vi "SubVI.vi"(5 "Durchläufegesamt":i32, 6 "Array 2":string[](array[string])=array[20229 elements], 10 "search String":string=".vi") -> (0 "Numerisches Element":i32, 2 "#found":i32, 3 "Array":string[](array[string]), 4 "work done analyse":dbl(slide) scale=0.0..100.0)   [LabVIEW 2009]
panel:
  out "search":string[](array[string])
  out "found":string[](array[string])
  out "Array 7":i32[](array[numeric])
  out "Array 6":string[](array[string])
  out "Array 5":bool[](array[boolean])
  out "zwischenerg":string[](array[string])
  out "Array 3":bool[](array[boolean])
  out "Elementindex":i32
  out "Zeilenanzahl":i32
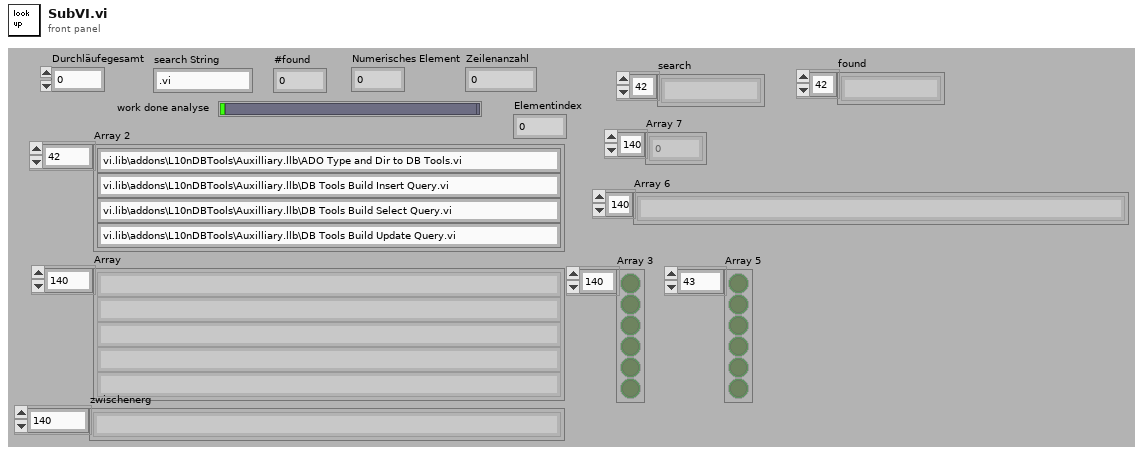
[diagram p1: front panel]
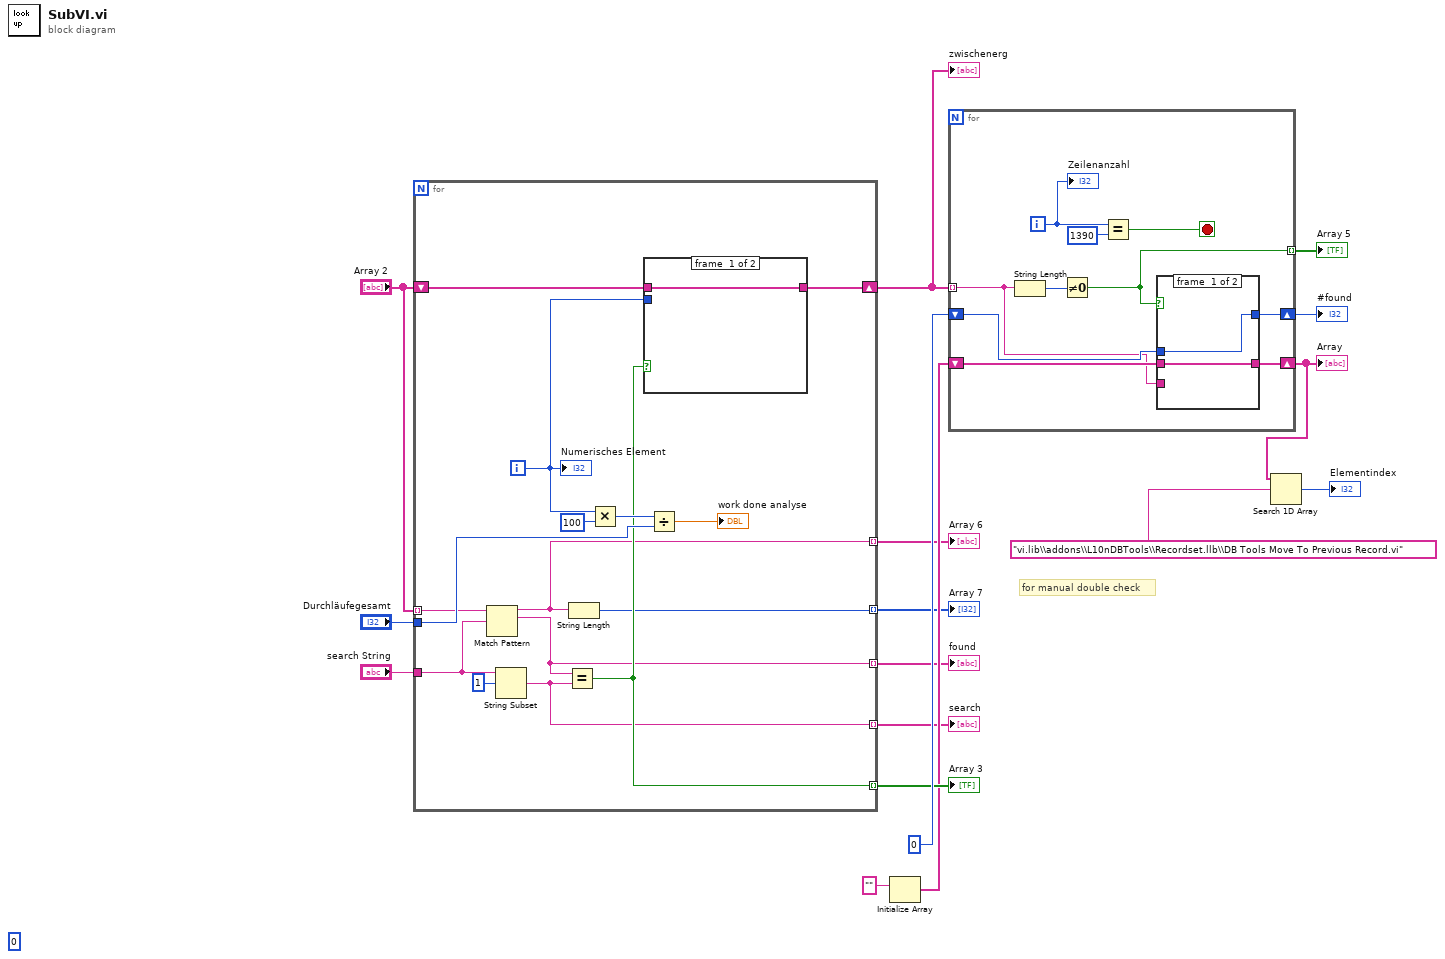
[diagram p0: block diagram]
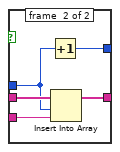
[diagram p2: hidden frame]
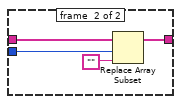
[diagram p3: hidden frame]
diagram:
  (unwired) 0
  # "for manual double check"
  n1 = for {
    tunnel: "Durchläufegesamt" -> [w30]
    tunnel: "Array 2" -> [w28] mode=indexing
    shift-right: [w26] -> w7
    shift-left: "Array 2" -> [w27]
    tunnel: "search String" -> [w20]
    tunnel: [w24] -> w12 mode=indexing
    tunnel: [w23] -> w6 mode=indexing
    tunnel: [w22] -> w5 mode=indexing
    tunnel: [w21] -> w3 mode=indexing
    tunnel: [w18] -> w2 mode=indexing
    i -> [w25]
    n2 = Match Pattern(string=w28, regular expression=w20) -> (before substring=w23:string, match substring=w21:string)  [unwired: 3 out]
    n3 = String Subset(string=w20, offset (0)=1 ("Offset (0)")) -> (substring=w18:string)  [unwired: 1 out]
    n4 = Equal?(x=w21, y=w18) -> (x = y?=w24:bool)
    n5 = String Length(string=w23) -> (length=w22:i32)
    n6 = Multiply(x=w25, y=100) -> (x*y=w32:i32)
    n7 = case shown="True" w24 {
      tunnel: w27 -> [w33 w37]
      tunnel: [w33 w36] -> w26
      tunnel: w25 -> [_ w35]
      frame #0 {
      }
      frame #1 {
        n8 = Replace Array Subset(array=w37, new element="", index=w35) -> (w36:string[])
      }
    }
    n9 = Divide(x=w32, y=w30) -> (x/y=→"work done analyse":dbl)
    "Numerisches Element" <- w25
  }
  "Array 3" <- w12
  "zwischenerg" <- w7
  "Array 6" <- w6
  "Array 7" <- w5
  "found" <- w3
  "search" <- w2
  n10 = Initialize Array("") -> (w9:string[])  [unwired: 1 out]
  n11 = for {
    tunnel: w7 -> [w41] mode=indexing
    shift-right: [w46] -> w1
    shift-left: w9 -> [w47]
    shift-right: [w44] -> w11
    shift-left: 0 -> [w43]
    tunnel: [w42] -> w8 mode=indexing
    i -> [w40]
    stop <- w38 stop-if-true
    n12 = String Length(string=w41) -> (length=w45:i32)
    n13 = Not Equal To 0?(x=w45) -> (x != 0?=w42:bool)
    n14 = Equal?(x=w40, y=1390) -> (x = y?=w38:bool)
    n15 = case shown="True" w42 {
      tunnel: w47 -> [w49 w54]
      tunnel: w41 -> [_ w51]
      tunnel: [w49 w53] -> w46
      tunnel: [w48 w52] -> w44
      tunnel: w43 -> [w48 w50]
      frame #0 {
      }
      frame #1 {
        n16 = Increment(x=w50) -> (x+1=w52:i32)
        n17 = Insert Into Array(array=w54, index=w50, new element=w51) -> (w53:string[])
      }
    }
    "Zeilenanzahl" <- w40
  }
  "Array" <- w1
  "#found" <- w11
  "Array 5" <- w8
  n18 = Search 1D Array(1D array=w1, element="vi.lib\\addons\\L10nDBTools\\Recordset.llb\\DB Tools Move To Previous Record.vi") -> (index of element=→"Elementindex":i32)  [unwired: 1 out]
